vi "Trajectory Box Monitor.vi"() -> ()   [LabVIEW 2017]
uses:
  TCP/TCP Engine/Controls/RT- Queue States.ctl
  TCP/TCP Host/Controls/Control - Testscreen.ctl
  Controls/Testscreen_Input cluster.ctl
  <vilib>/addons/database/Connection.llb/Conn ObjectReference.ctl
  Controls/Network_states.ctl
  TCP/TCP Engine/TCP/TCP - Driver Control.ctl
  Variable/Global 1.vi
  <vilib>/addons/database/Connection.llb/DB Tools Open Connec (String).vi
  <vilib>/addons/database/NI_Database_API.lvlib
panel:
  out "error out":errorcluster
  out "array":string[](array[string])
  out "Test Running":bool
  in  "DataLog Duration":string="00:01:27"
  in  "Exit":bool
  in  "Report":bool
  in  "Settings":bool
  in  "Test Screen":bool
  in  "ID Status":string
  in  "?":enum32{"Option A", "Option B"}(tab)
  in  "Test Profile":T1(array[cluster])=[{"Ram Up Time"=10.0, "Hold Time"=5.0, "Ramp Down"=10.0, "Concentration Value"=25.0}, {"Ram Up Time"=15.0, "Hold Time"=10.0, "Ramp Down"=5.0, "Concentration Value"=35.0}, {"Ram Up Time"=0.0, "Hold Time"=0.0, "Ramp Down"=0.0, "Concentration Value"=0.0}]
  out "Profile Plotting":cluster{"X":dbl, "Y":dbl}[](graph)
  in  "Profile File Selection":u16(ring) items=["Test A", "Test B", "Test C"]
  in  "Iterations":dbl
  in  "Gas Selection":u16(ring) items=["Test A", "Test B", "Test C"]
  in  "Drive  2":string
  in  "Drive":string
  in  "IP Address":string
  in  "error in (no error)":errorcluster
  in  "Note":string
  in  "Tab- Main":enum32{"Settings", "Report", "Testscreen"}(tab)
  in  "Tab Control Testscreen 4":enum32{"Channel Mapping", "Test Settings"}(tab)
  in  "Channel Mapping":T2(array[cluster])
  in  "Sampling Frequency (Hz)":string="Trajectory"
  in  "Wifi Name":string="Trajectory"
  in  "Test Inactivity Time":dbl=30.0 format="%<%H:%M:%S>t"
  in  "Drive Path":path=path "D:/Trajectory Data"
  in  "cRIO IP Address":string="192.168.1.1"
  out "Test Time":dbl=1.0 format="%<%H:%M:%S>t"
  in  "Save Test Settings":bool
  in  "Tab Control Testscreen 5":enum32{"Report", "Detailed Report"}(tab)
  in  "Fetch Report":bool
  in  "To Date & Time":timestamp format="%<%x>T"
  in  "From Date & Time":timestamp format="%<%x>T"
  out "Report Data":i32(listbox)
  in  "Test Stop Time :":string="12:59:05"
  in  "Tab Control Testscreen 6":enum32{"Data", "Histogram"}(tab)
  in  "Report Data 2":i32(listbox)
  out "XY Graph 3":cluster{i32, "Numeric":u16}[](graph)
  in  "ID Status :":string="00068OK"
  in  "ID :":string="Trajectory"
  in  "Angle :":string="Multi"
  in  "Flow :":string="Flow"
  in  "Material :":string="Cole"
  in  "Furnace :":string="G Furnace"
  in  "Test Start Time:":string="12:59:05"
  in  "Date :":string="02/07/2021"
  out "Date":string
  in  "Tab- Main 2":T3(tab)
  in  "Test details":T4={"Furnace"="Furnace A", "Material"="Coke", "Angle"="Multi Angle", "ID"="Trajectory 9", "Flowrate"="Flow", "Test Name"="Coke Burn", "Tested By"="Anirban"}
  in  "Save Test Info":bool
  out "Data Logging Path":path
  in  "Probe 2":bool[](array[boolean])=[TRUE, FALSE, FALSE, FALSE, TRUE, FALSE, FALSE, FALSE, FALSE, FALSE, FALSE, FALSE, FALSE, FALSE, FALSE, FALSE, FALSE, FALSE, FALSE, FALSE, FALSE, FALSE, FALSE, FALSE, FALSE, FALSE, FALSE, FALSE, FALSE, FALSE, FALSE, FALSE, FALSE, FALSE, FALSE, FALSE, FALSE, FALSE, FALSE, FALSE, FALSE, FALSE, FALSE, FALSE, FALSE, FALSE, FALSE, FALSE, FALSE, FALSE, FALSE, FALSE, FALSE, FALSE, FALSE, FALSE, FALSE, FALSE, FALSE, FALSE]
  in  "Probe":bool[](array[boolean])
  in  "Probe 3":bool[](array[boolean])=[TRUE, FALSE, FALSE, FALSE, TRUE, FALSE, FALSE, FALSE, FALSE, FALSE, FALSE, FALSE, FALSE, FALSE, FALSE, FALSE, FALSE, FALSE, FALSE, FALSE, FALSE, FALSE, FALSE, FALSE, FALSE, FALSE, FALSE, FALSE, FALSE, FALSE, FALSE, FALSE, FALSE, FALSE, FALSE, FALSE, FALSE, FALSE, FALSE, FALSE, FALSE, FALSE, FALSE, FALSE, FALSE, FALSE, FALSE, FALSE, FALSE, FALSE, FALSE, FALSE, FALSE, FALSE, FALSE, FALSE, FALSE, FALSE, FALSE, FALSE]
  out "XY Graph":cluster{i32, "Numeric":i32}[](graph)
  in  "Setup":bool
  out "Datalog Duration":dbl format="%<%H:%M:%S>t"
  in  "Disk Space Host":string="Trajectory 9"
  in  "Disk Space cRIO":string="Trajectory 9"
  in  "Calibrations":bool
  in  "Alarms":i32(listbox)
  out "Wifi":bool=TRUE
  out "Logging 3":bool=TRUE
  in  "Start Test":bool
  in  "Stop Test":bool
  out "Message":string="Acquiring Data"
  # "Test Setup Setting"
  # "Trajectory Box Monitor System"
  # "Trajectory Box Monitor"
  # "1"
  # "5"
  # "10"
  # "15"
  # "20"
  # "41"
  # "45"
  # "50"
  # "55"
  # "60"
  # "21"
  # "25"
  # "30"
  # "40"
  # "35"
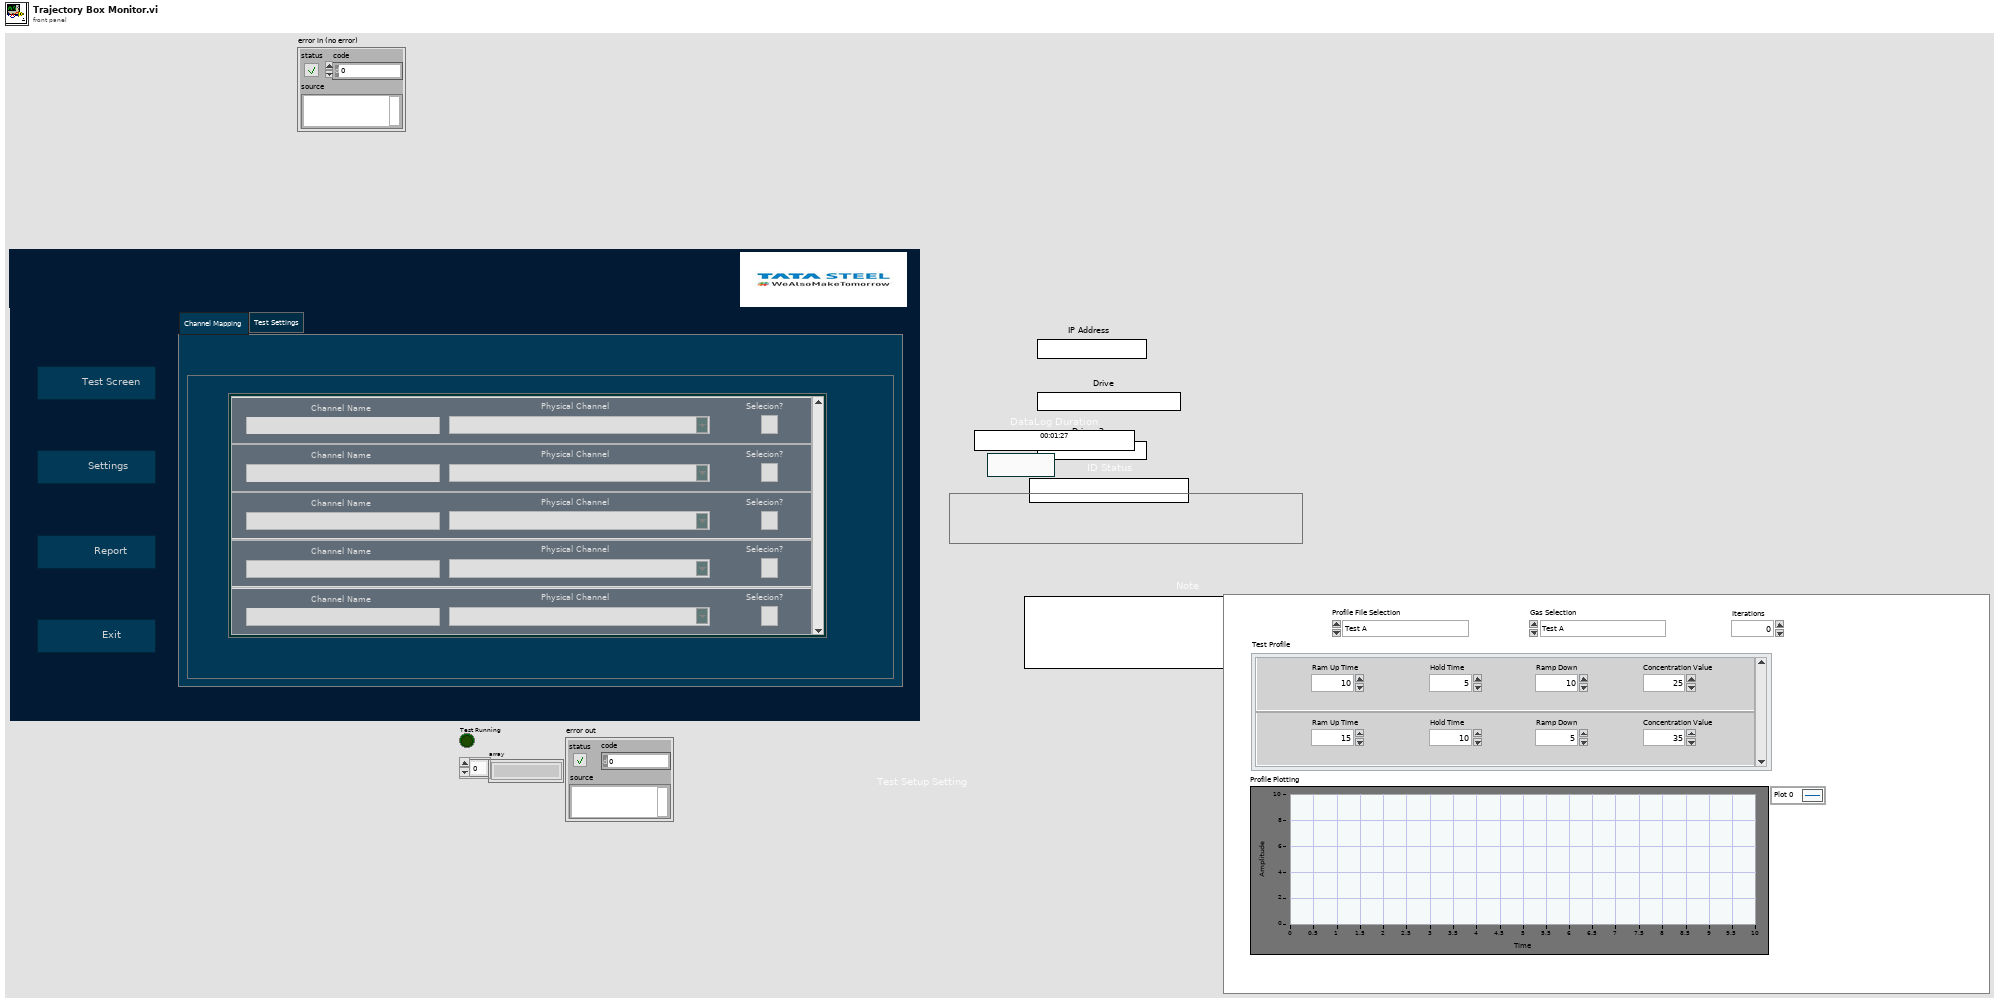
[diagram p1: front panel]
types:
  T1 = cluster{"Ram Up Time":dbl, "Hold Time":dbl, "Ramp Down":dbl, "Concentration Value":dbl}[]
  T2 = cluster{"Channel Name":string, " Physical Channel":tag, "Selecion?":bool}[]
  T3 = enum32{"Test Information", "Sensor Status", "Histogram", "Info", "Software Log"}
  T4 = cluster{"Furnace":string, "Material":string, "Angle":string, "ID":string, "Flowrate":string, "Test Name":string, "Tested By":string}
  T5 = typedef "Network_states.ctl" = enum16{"Connect", "Transfer Files", "Close"}
  T6 = typedef "Testscreen_Input cluster.ctl" = cluster{"Message":string, "Histogram Data":i32[], "Timer 1":u32, "Test Running":bool, "connection reference":T7}
  T7 = typedef "NI_Database_API.lvlib/Conn ObjectReference.ctl" = refnum<k1>
  T8 = typedef "Control - Testscreen.ctl" = enum16{"No Event", "Init", "Download Files", "Test Running", "Update Test Results", "Machine Unhealthy", "Autotest Started", "Test Aborted", "Sequence Complete", "Update Sensor Data", "Log File Available", "Machine Mode", "Aux Logging Started", "Aux File Saved", "Get PID Values", "View Report", "Exit", "Wait", "Abort", "Copy Log File", "Send Test Details"}
  T9 = typedef "RT- Queue States.ctl" = enum16{"Initialize", "Enqueue", "Enqueue Priority", "Dequeue", "Flush", "Destroy"}
  T10 = cluster{"Test details":cluster{"Furnace":string, "Material":string, "Angle":string, "ID":string, "Flowrate":string, "Test Name":string, "Tested By":string}, "Datalog Duration":dbl}
  T11 = typedef "TCP - Driver Control.ctl" = enum16{"Test Settings", "Boolean Commands", "Test Results", "Send Test Details"}
  T12 = cluster{"Channel Name":string, " Physical Channel":tag, "Selecion?":bool}
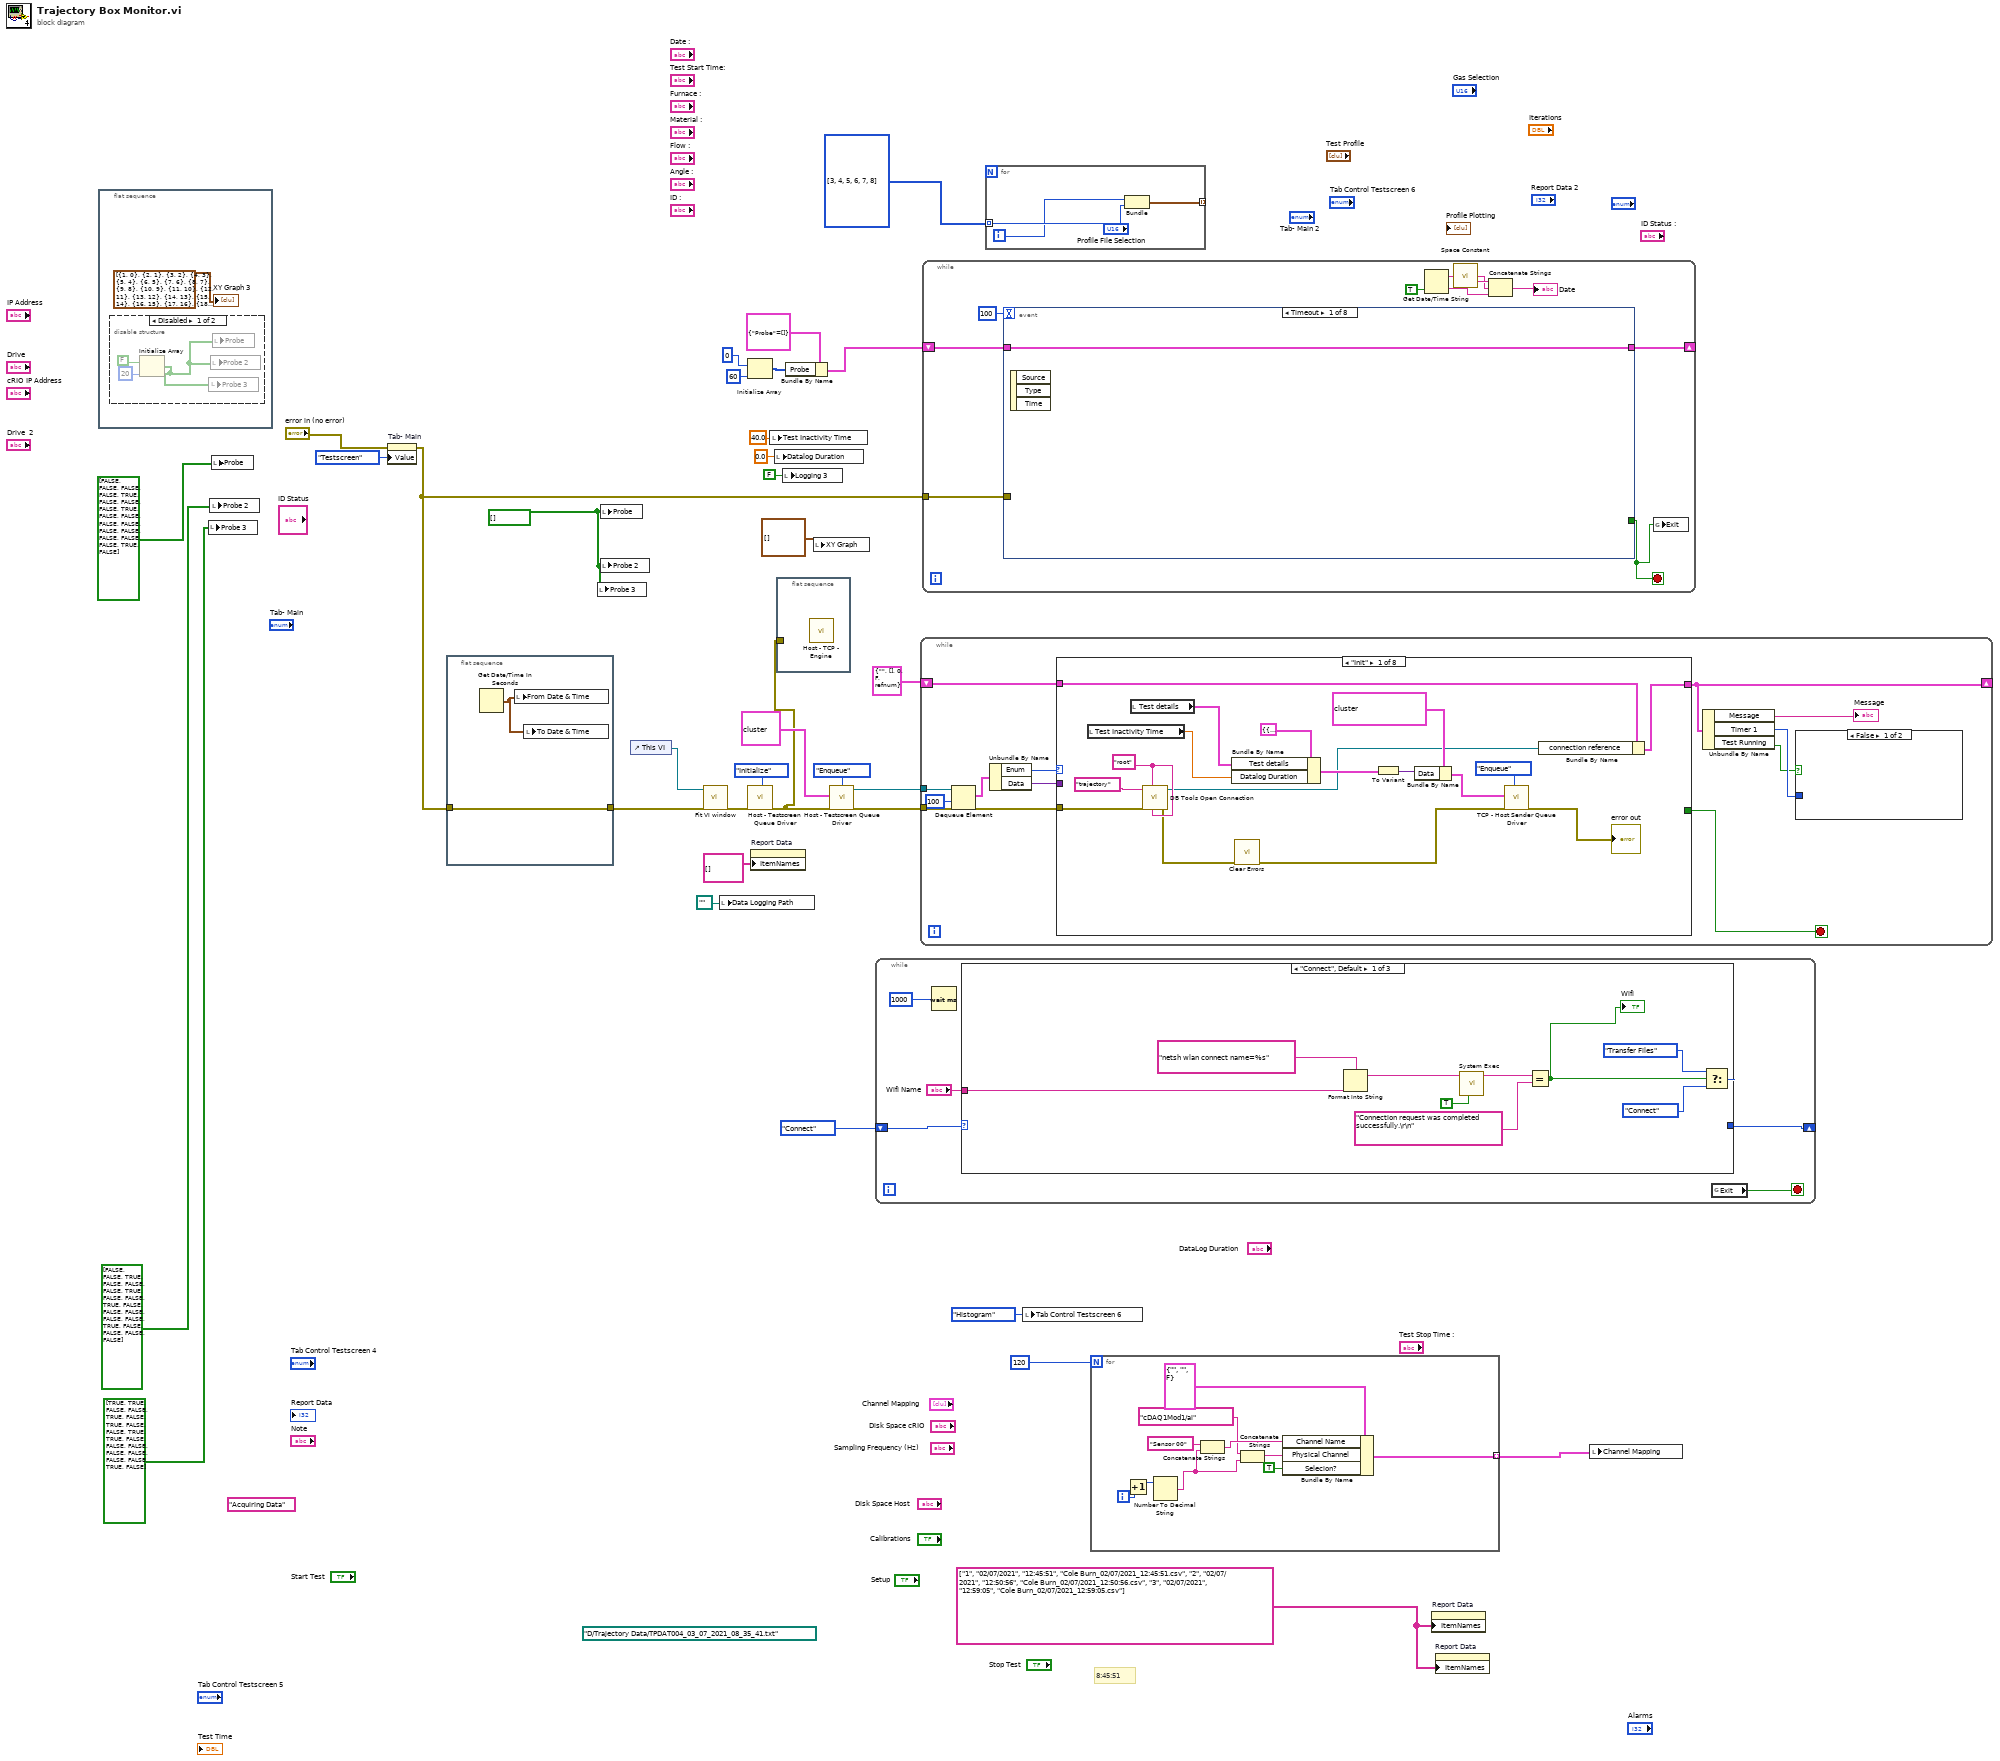
[diagram p0: block diagram]
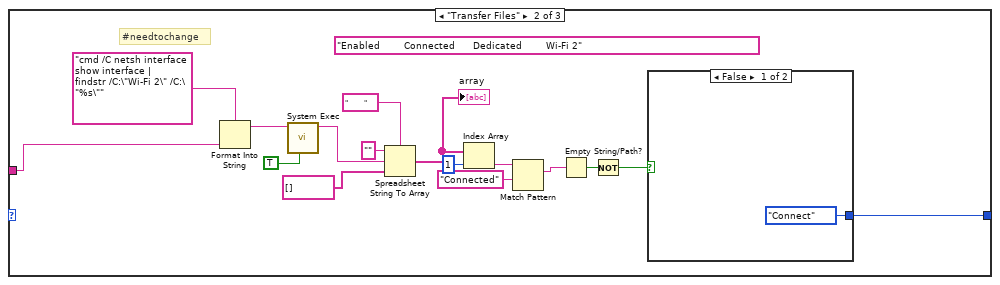
[diagram p2: hidden frame]
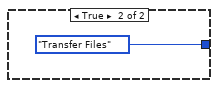
[diagram p3: hidden frame]
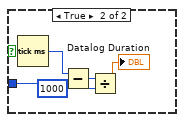
[diagram p5: hidden frame]
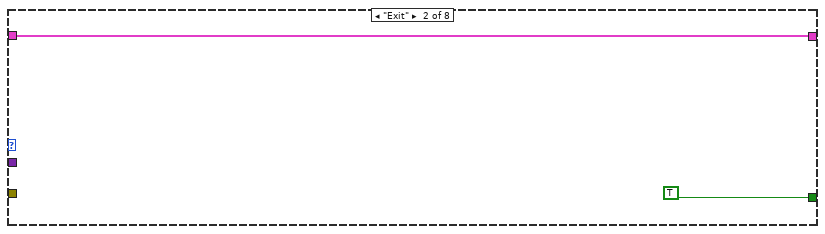
[diagram p6: hidden frame]
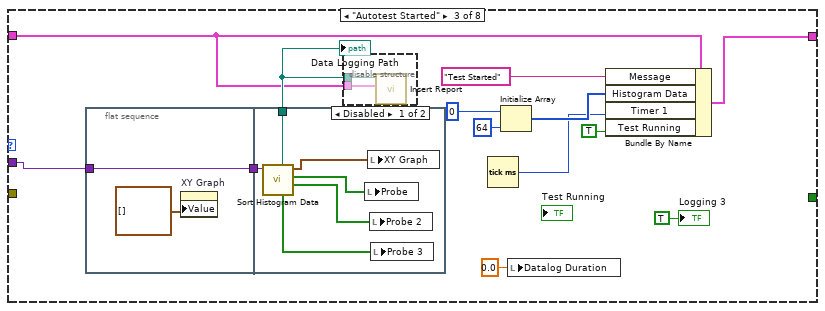
[diagram p7: hidden frame]
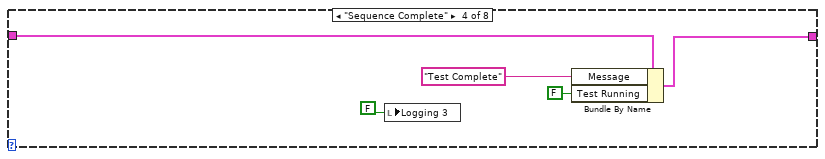
[diagram p9: hidden frame]
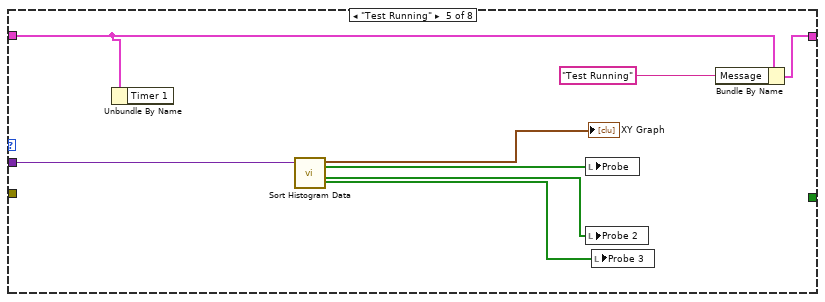
[diagram p10: hidden frame]
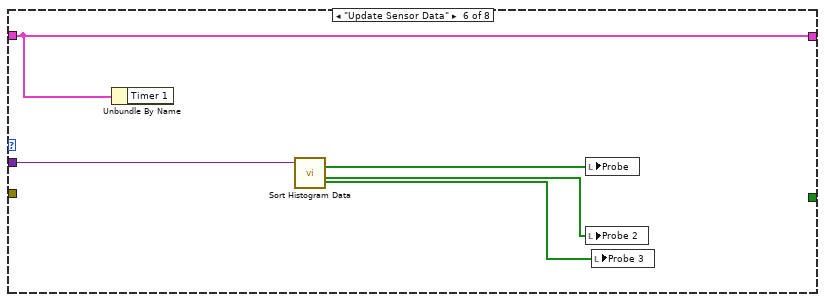
[diagram p11: hidden frame]
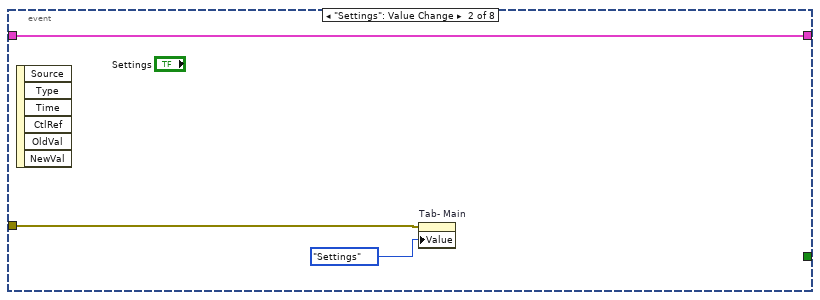
[diagram p15: hidden frame]
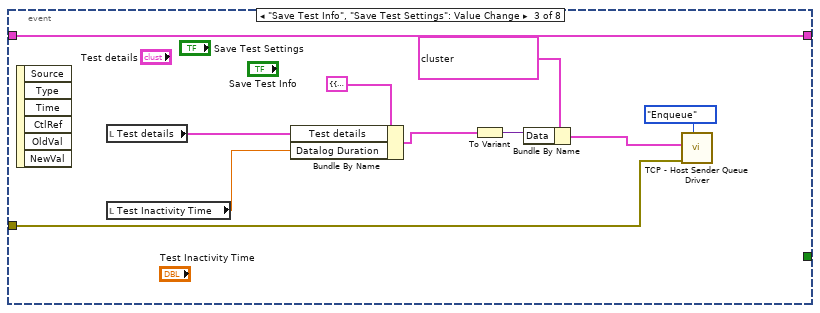
[diagram p16: hidden frame]
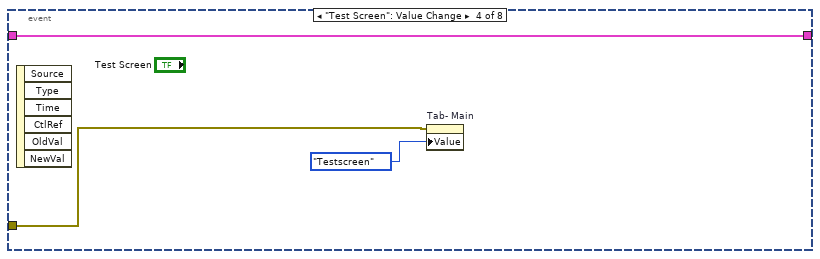
[diagram p17: hidden frame]
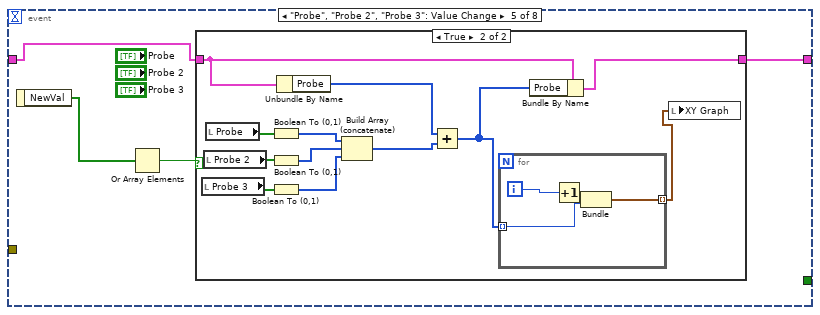
[diagram p18: hidden frame]
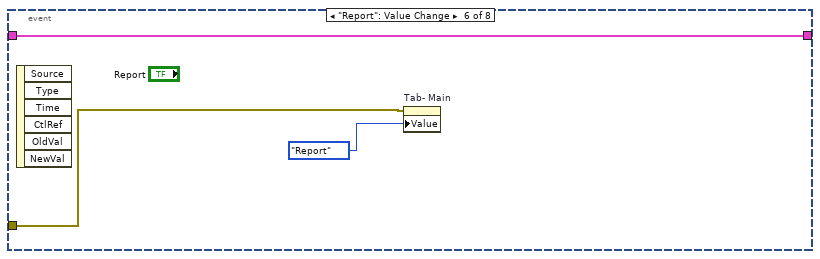
[diagram p20: hidden frame]
diagram:
  w13 = bool[] [] ("Probe")
  w20 = string[][] [["1", "02/07/2021", "12:45:51", "Cole Burn_02/07/2021_12:45:51.csv"], ["2", "02/07/2021", "12:50:56", "Cole Burn_02/07/2021_12:50:56.csv"], ["3", "02/07/2021", "12:59:05", "Cole Burn_02/07/2021_12:59:05.csv"]] ("Item Names")
  (unwired) path "D:/Trajectory Data/TPDAT004_03_07_2021_08_35_41.txt" ("Data Logging Path")
  (unwired) "Acquiring Data" ("Message")
  # "8:45:51"
  n1 = flat-sequence {
    frame #0 {
      n2 = disable-structure shown="Disabled" {
        frame Disabled {
          n3 = Initialize Array(FALSE ("Boolean"), 20 ("dimension size")) -> (w36:bool[])
          n4 = local write "Probe 3"(w36) -> ()
          n5 = local write "Probe 2"(w36) -> ()
          n6 = local write "Probe"(w36) -> ()
        }
        frame Enabled {
        }
      }
      "XY Graph 3" <- cluster{i32, "Numeric":u16}[] [{1, "Numeric"=0}, {2, "Numeric"=1}, {3, "Numeric"=2}, {4, "Numeric"=3}, {5, "Numeric"=4}, {6, "Numeric"=5}, {7, "Numeric"=6}, {8, "Numeric"=7}, {9, "Numeric"=8}, {10, "Numeric"=9}, {11, "Numeric"=10}, {12, "Numeric"=11}, {13, "Numeric"=12}, {14, "Numeric"=13}, {15, "Numeric"=14}, {16, "Numeric"=15}, {17, "Numeric"=16}, {18, "Numeric"=17}, {19, "Numeric"=18}, {20, "Numeric"=19}, {21, "Numeric"=20}, {22, "Numeric"=21}, {23, "Numeric"=22}, {24, "Numeric"=23}, {25, "Numeric"=24}, {26, "Numeric"=25}, {27, "Numeric"=26}, {28, "Numeric"=27}, {29, "Numeric"=28}, {30, "Numeric"=29}, {30, "Numeric"=29}, {31, "Numeric"=28}, {32, "Numeric"=27}, {33, "Numeric"=26}, {34, "Numeric"=25}, {35, "Numeric"=24}, {36, "Numeric"=23}, {37, "Numeric"=22}, {38, "Numeric"=21}, {39, "Numeric"=20}, {40, "Numeric"=19}, {41, "Numeric"=18}, {42, "Numeric"=17}, {43, "Numeric"=16}, {44, "Numeric"=15}, {45, "Numeric"=14}, {46, "Numeric"=13}, {47, "Numeric"=12}, {48, "Numeric"=11}, {49, "Numeric"=10}, {50, "Numeric"=9}, {51, "Numeric"=8}, {52, "Numeric"=7}, {53, "Numeric"=6}, {54, "Numeric"=5}, {55, "Numeric"=4}, {56, "Numeric"=3}, {57, "Numeric"=2}, {58, "Numeric"=1}, {59, "Numeric"=0}] ("appended array 2")
    }
  }
  n7 = local write "Probe 3"(bool[] [TRUE, TRUE, FALSE, FALSE, TRUE, FALSE, TRUE, FALSE, FALSE, TRUE, TRUE, FALSE, FALSE, FALSE, FALSE, FALSE, FALSE, FALSE, TRUE, FALSE] ("Probe")) -> ()
  n8 = local write "Probe 2"(bool[] [FALSE, FALSE, TRUE, FALSE, FALSE, FALSE, TRUE, FALSE, FALSE, TRUE, FALSE, FALSE, FALSE, FALSE, FALSE, TRUE, FALSE, FALSE, FALSE, FALSE] ("Probe")) -> ()
  n9 = local write "Probe"(bool[] [FALSE, FALSE, FALSE, FALSE, TRUE, FALSE, FALSE, FALSE, TRUE, FALSE, FALSE, FALSE, FALSE, FALSE, FALSE, FALSE, FALSE, FALSE, TRUE, FALSE] ("Probe")) -> ()
  n10 = property on="Tab- Main" class="TabCtl (strict)"(error in="error in (no error)", "Value"=enum32{"Settings", "Report", "Testscreen"}."Testscreen" ("Tab- Main")) -> (error out=w4:errorcluster)  [unwired: 1 in, 1 out]
  n11 = flat-sequence {
    tunnel: [w40] -> w3
    tunnel: w4 -> [w40]
    frame #0 {
      n12 = Get Date/Time In Seconds() -> (seconds since 1Jan1904=w39:timestamp)
      n13 = local write "From Date & Time"(w39) -> ()
      n14 = local write "To Date & Time"(w39) -> ()
    }
  }
  n15 = local write "Probe 3"(w13) -> ()
  n16 = local write "Probe"(w13) -> ()
  n17 = local write "Probe 2"(w13) -> ()
  n18 = control-ref of="This VI"() -> (w9:refnum<vi>)
  n19 = call "Fit VI window.vi"("error in (no error)"=w3, "VI Ref (calling VI)"=w9) -> ("error out"=w10:errorcluster)  [unwired: 9 in]
  n20 = local write "Data Logging Path"(path "" ("Data Logging Path")) -> ()
  n21 = Initialize Array(0 ("Numeric"), 60 ("dimension size")) -> (w30:i32[])
  n22 = call "Host - Testscreen Queue Driver.vi"("Cases"=RT-_Queue_States."Initialize", "error in (no error)"=w10) -> ("error out"=w1:errorcluster)  [unwired: 7 in, 2 out]
  n23 = property on="Report Data" class="MCListbox (strict)"("ItemNames"=string[][] [] ("Item Names")) -> ()  [unwired: 2 in, 2 out]
  n24 = local write "Test Inactivity Time"(40.0 ("Datalog Duration")) -> ()
  n25 = local write "Datalog Duration"(0.0 ("Datalog Duration")) -> ()
  n26 = flat-sequence {
    tunnel: w1 -> [_]
    frame #0 {
      n27 = call "Host - TCP - Engine.vi"() -> ()  [unwired: 12 in]
    }
  }
  n28 = local write "Logging 3"(FALSE ("Logging 3")) -> ()
  n29 = Bundle By Name(cluster=cluster{"Probe":i32[]} {"Probe"=[]}, "Probe"=w30) -> (w28:cluster{"Probe":i32[]})
  n30 = local write "XY Graph"(cluster{i32, "Numeric":i32}[] [] ("XY Graph")) -> ()
  n31 = call "Host - Testscreen Queue Driver.vi"("Cases"=RT-_Queue_States."Enqueue", "error in (no error)"=w1, "Element In"=cluster{"Data":variant, "Enum":T8} {"Data"=variant, "Enum"=enum."Init"}) -> ("error out"=w15:errorcluster, "queue out"=w17:refnum<queue>)  [unwired: 6 in, 1 out]
  n32 = while {
    shift-right: [w43] -> _
    shift-left: Network_states."Connect" -> [w44]
    stop <- w45 stop-if-true
    n33 = Wait (ms)(milliseconds to wait=u32 1000) -> ()  [unwired: 1 out]
    n34 = case shown="\"Connect\", Default" w44 {
      tunnel: [w48 w56 _] -> w43
      tunnel: "Wifi Name" -> [w47 w68 _]
      frame "Connect", Default {
        n35 = Format Into String(format string="netsh wlan connect name=%s" ("command line"), w47) -> (resulting string=w51:string)  [unwired: 2 in, 1 out]
        n36 = call <vilib>:"System Exec.vi"("run minimized? (F)"=TRUE, "command line"=w51) -> ("standard output"=w54:string)  [unwired: 6 in, 3 out]
        n37 = Equal?(x=w54, y="Connection request was completed successfully.\r\n") -> (x = y?=w46:bool)
        "Wifi" <- w46
        n38 = Select(t=Network_states."Transfer Files", s=w46, f=Network_states."Connect") -> (s? t:f=w48:T5)
      }
      frame "Transfer Files" {
        (unwired) "Enabled        Connected      Dedicated        Wi-Fi 2" ("format string")
        # "#needtochange"
        n39 = Format Into String(format string="cmd /C netsh interface show interface | findstr /C:\"Wi-Fi 2\" /C:\"%s\"" ("command line"), w68) -> (resulting string=w70:string)  [unwired: 2 in, 1 out]
        n40 = call <vilib>:"System Exec.vi"("run minimized? (F)"=TRUE, "command line"=w70) -> ("standard output"=w66:string)  [unwired: 6 in, 3 out]
        n41 = Spreadsheet String To Array(delimiter (Tab)="        ", format string="", spreadsheet string=w66, array type (2D Dbl)=string[] []) -> (array=w63:string[])
        "array" <- w63
        n42 = Index Array(array=w63, index=1) -> (element=w61:string)
        n43 = Match Pattern(string=w61, regular expression="Connected") -> (match substring=w59:string)  [unwired: 1 in, 3 out]
        n44 = Empty String/Path?(string/path=w59) -> (empty?=w58:bool)
        n45 = Not(x=w58) -> (.not. x?=w57:bool)
        n46 = case shown="False" w57 {
          tunnel: [Network_states."Connect" Network_states."Transfer Files"] -> w56
          frame False {
          }
          frame True {
          }
        }
      }
      frame "Close" {
      }
    }
    n47 = global read "Global 1.vi" "Exit"() -> (w45:bool)
  }
  n48 = while {
    tunnel: w15 -> [w84]
    tunnel: w17 -> [w85]
    shift-right: [w79] -> _
    shift-left: T6 {"Message"="", "Histogram Data"=[], "Timer 1"=0, "Test Running"=FALSE, "connection reference"=refnum} -> [w80]
    stop <- w86 stop-if-true
    n49 = Dequeue Element(queue=w85, timeout in ms (-1)=100, error in (no error)=w84) -> (element=w82:cluster{"Data":variant, "Enum":T8}, error out=w83:errorcluster)  [unwired: 2 out]
    n50 = Unbundle By Name(w82) -> ("Enum"=w81:T8, "Data"=w77:variant)
    n51 = case shown="\"Init\"" w81 {
      tunnel: w83 -> [w98 _ _ _ _ _ _ _]
      tunnel: [_ TRUE _ _ _ _ _ _] -> w86
      tunnel: w80 -> [w95 w109 w111 w138 w139 w147 w152 w153]
      tunnel: [w94 w109 w122 w136 w142 w147 w152 w153] -> w79
      tunnel: w77 -> [_ _ w118 _ w146 w151 _ _]
      frame "Init" {
        w99 = "root" ("userID")
        n52 = local read "Test Inactivity Time"() -> (w101:dbl)
        n53 = local read "Test details"() -> (w103:T4)
        n54 = call-poly <vilib>:"DB Tools Open Connection.vi"("password"=w99, "userID"=w99, "error in (no error)"=w98, "connection information"="trajectory") -> ("error out"=w97:errorcluster, "connection reference"=w96:T7)  [unwired: 4 in]
        n55 = Bundle By Name(cluster=T10 {"Test details"={"Furnace"="Furnace A", "Material"="Aluminium", "Angle"="Multi Angle", "ID"="Trajectory 9", "Flowrate"="Flow", "Test Name"="Coke Burn", "Tested By"="Anirban"}, "Datalog Duration"=0.0}, "Test details"=w103, "Datalog Duration"=w101) -> (w102:T10)
        n56 = call <vilib>:"Clear Errors.vi"("error in (no error)"=w97) -> ("error out"=w93:errorcluster)  [unwired: 5 in, 1 out]
        n57 = To Variant(anything=w102) -> (Variant=w105:variant)
        n58 = Bundle By Name(cluster=cluster{"Data":variant, "State":T11} {"Data"=variant, "State"=enum."Send Test Details"} ("Element In"), "Data"=w105) -> (w108:cluster{"Data":variant, "State":T11})
        n59 = call "TCP - Host Sender Queue Driver.vi"("Cases"=RT-_Queue_States."Enqueue", "error in (no error)"=w93, "Element In"=w108) -> ("error out"=→"error out":errorcluster)  [unwired: 6 in, 2 out]
        n60 = Bundle By Name(cluster=w95, "connection reference"=w96) -> (w94:T6)
      }
      frame "Exit" {
      }
      frame "Autotest Started" {
        n61 = flat-sequence {
          tunnel: w118 -> [w127]
          tunnel: [w127] -> w117
          tunnel: w117 -> [w133]
          tunnel: [w128] -> w112
          frame #0 {
            n62 = property on="XY Graph" class="XYGraph (strict)"("Value"=cluster{i32, "Numeric":u16}[] [] ("XY Graph")) -> ()  [unwired: 2 in, 2 out]
          }
          frame #1 {
            n63 = call "Sort Histogram Data.vi"("Data"=w133) -> ("Array 2"=w130:bool[], "Array 3"=w131:bool[], "XY Graph"=w132:cluster{i32, "Numeric":i32}[], "Array"=w129:bool[], "File Path"=w128:path)  [unwired: 6 in]
            n64 = local write "Probe"(w131) -> ()
            n65 = local write "XY Graph"(w132) -> ()
            n66 = local write "Probe 2"(w130) -> ()
            n67 = local write "Probe 3"(w129) -> ()
          }
        }
        n68 = disable-structure shown="Disabled" {
          disable-tunnel: w112 -> [w125 _]
          disable-tunnel: w111 -> [w124 _]
          frame Disabled {
            n69 = call "Insert Report.vi"("Cluster"=w124, "Path"=w125) -> ()  [unwired: 9 in, 1 out]
          }
          frame Enabled {
          }
        }
        n70 = Tick Count (ms)() -> (millisecond timer value=w116:u32)
        n71 = Initialize Array(0, 64 ("dimension size")) -> (w119:i32[])
        n72 = local write "Datalog Duration"(0.0 ("Datalog Duration")) -> ()
        n73 = Bundle By Name(cluster=w111, "Message"="Test Started", "Histogram Data"=w119, "Timer 1"=w116, "Test Running"=TRUE) -> (w122:T6)
        "Data Logging Path" <- w112
        "Logging 3" <- TRUE ("Logging 3")
      }
      frame "Sequence Complete" {
        n74 = local write "Logging 3"(FALSE ("Logging 3")) -> ()
        n75 = Bundle By Name(cluster=w138, "Message"="Test Complete", "Test Running"=FALSE) -> (w136:T6)
      }
      frame "Test Running" {
        n76 = Unbundle By Name(w139) -> ()  [unwired: 1 out]
        n77 = call "Sort Histogram Data.vi"("Data"=w146) -> ("Array 2"=w144:bool[], "Array 3"=w145:bool[], "XY Graph"=→"XY Graph":cluster{i32, "Numeric":i32}[], "Array"=w143:bool[])  [unwired: 6 in, 1 out]
        n78 = local write "Probe"(w145) -> ()
        n79 = local write "Probe 2"(w144) -> ()
        n80 = local write "Probe 3"(w143) -> ()
        n81 = Bundle By Name(cluster=w139, "Message"="Test Running") -> (w142:T6)
      }
      frame "Update Sensor Data" {
        n82 = Unbundle By Name(w147) -> ()  [unwired: 1 out]
        n83 = call "Sort Histogram Data.vi"("Data"=w151) -> ("Array 2"=w149:bool[], "Array 3"=w150:bool[], "Array"=w148:bool[])  [unwired: 6 in, 2 out]
        n84 = local write "Probe"(w150) -> ()
        n85 = local write "Probe 2"(w149) -> ()
        n86 = local write "Probe 3"(w148) -> ()
      }
      frame "No Event", Default {
      }
      frame "Update Test Results" {
      }
    }
    n87 = Unbundle By Name(w79) -> ("Message"=→"Message":string, "Timer 1"=w76:u32, "Test Running"=w75:bool)
    n88 = case shown="False" w75 {
      tunnel: w76 -> [_ w90]
      frame False {
      }
      frame True {
        n89 = Tick Count (ms)() -> (millisecond timer value=w91:u32)
        n90 = Subtract(x=w91, y=w90) -> (x-y=w89:u32)
        n91 = Divide(x=w89, y=u32 1000) -> (x/y=→"Datalog Duration":dbl)
      }
    }
  }
  n92 = while {
    tunnel: w4 -> [w163]
    shift-right: [w161] -> _
    shift-left: w28 -> [w162]
    stop <- w154 stop-if-true
    n93 = event shown="[0] Timeout" {
      selector: _ -> [_ _ _ _ _ _ _ _]
      dyn-events: _ -> [_ _ _ _ _ _ _ _]
      timeout: 100 -> [_ _ _ _ _ _ _ _]
      tunnel: [_ _ _ _ _ _ TRUE _] -> w154
      tunnel: w163 -> [_ w167 w168 w180 _ w204 w205 _]
      tunnel: w162 -> [w164 w166 w177 w179 w182 w203 w208 w212]
      tunnel: [w164 w166 w177 w179 w181 w203 w208 w212] -> w161
      event Timeout {
        n94 = event-data() -> ()  [unwired: 1 in, 3 out]
      }
      event "Settings": Value Change {
        n95 = event-data() -> ()  [unwired: 1 in, 6 out]
        n96 = property on="Tab- Main" class="TabCtl (strict)"(error in=w167, "Value"=enum32{"Settings", "Report", "Testscreen"}."Settings" ("Tab- Main")) -> ()  [unwired: 1 in, 2 out]
      }
      event "Save Test Info", "Save Test Settings": Value Change {
        n97 = event-data() -> ()  [unwired: 1 in, 6 out]
        n98 = local read "Test details"() -> (w174:T4)
        n99 = local read "Test Inactivity Time"() -> (w176:dbl)
        n100 = Bundle By Name(cluster=T10 {"Test details"={"Furnace"="Furnace A", "Material"="Aluminium", "Angle"="Multi Angle", "ID"="Trajectory 9", "Flowrate"="Flow", "Test Name"="Coke Burn", "Tested By"="Anirban"}, "Datalog Duration"=0.0}, "Test details"=w174, "Datalog Duration"=w176) -> (w175:T10)
        n101 = To Variant(anything=w175) -> (Variant=w172:variant)
        n102 = Bundle By Name(cluster=cluster{"Data":variant, "State":T11} {"Data"=variant, "State"=enum."Send Test Details"} ("Element In"), "Data"=w172) -> (w169:cluster{"Data":variant, "State":T11})
        n103 = call "TCP - Host Sender Queue Driver.vi"("Cases"=RT-_Queue_States."Enqueue", "error in (no error)"=w168, "Element In"=w169) -> ()  [unwired: 6 in, 3 out]
      }
      event "Test Screen": Value Change {
        n104 = event-data() -> ()  [unwired: 1 in, 6 out]
        n105 = property on="Tab- Main" class="TabCtl (strict)"(error in=w180, "Value"=enum32{"Settings", "Report", "Testscreen"}."Testscreen" ("Tab- Main")) -> ()  [unwired: 1 in, 2 out]
      }
      event "Probe", "Probe 2", "Probe 3": Value Change {
        n106 = event-data() -> ("NewVal"=w184:bool[])  [unwired: 1 in]
        n107 = Or Array Elements(Boolean array=w184) -> (logical OR=w183:bool)
        n108 = case shown="True" w183 {
          tunnel: w182 -> [w185 w188]
          tunnel: [w185 w187] -> w181
          frame False {
          }
          frame True {
            n109 = local read "Probe 3"() -> (w195:bool[])
            n110 = local read "Probe 2"() -> (w196:bool[])
            n111 = local read "Probe"() -> (w197:bool[])
            n112 = Boolean To (0,1)(Boolean=w197) -> (0, 1=w194:i16[])
            n113 = Boolean To (0,1)(Boolean=w196) -> (0, 1=w193:i16[])
            n114 = Boolean To (0,1)(Boolean=w195) -> (0, 1=w192:i16[])
            n115 = Unbundle By Name(w188) -> ("Probe"=w191:i32[])
            n116 = Build Array (concatenate)(w194, w193, w192) -> (w190:i16[])
            n117 = Add(x=w191, y=w190) -> (x+y=w186:i32[])
            n118 = for {
              tunnel: [w201] -> w189 mode=indexing
              tunnel: w186 -> [w200] mode=indexing
              i -> [w199]
              n119 = Increment(x=w199) -> (x+1=w198:i32)
              n120 = Bundle(w198, w200) -> (w201:cluster{i32, i32})  [unwired: 1 in]
            }
            n121 = Bundle By Name(cluster=w188, "Probe"=w186) -> (w187:cluster{"Probe":i32[]})
            n122 = local write "XY Graph"(w189) -> ()
          }
        }
      }
      event "Report": Value Change {
        n123 = event-data() -> ()  [unwired: 1 in, 6 out]
        n124 = property on="Tab- Main" class="TabCtl (strict)"(error in=w204, "Value"=enum32{"Settings", "Report", "Testscreen"}."Report" ("Tab- Main")) -> ()  [unwired: 1 in, 2 out]
      }
      event "Exit": Value Change {
        n125 = event-data() -> ()  [unwired: 1 in, 6 out]
        n126 = call "Host - Testscreen Queue Driver.vi"("Cases"=RT-_Queue_States."Enqueue", "error in (no error)"=w205, "Element In"=cluster{"Data":variant, "Enum":T8} {"Data"=variant, "Enum"=enum."Exit"}) -> ()  [unwired: 6 in, 3 out]
      }
      event "Fetch Report": Value Change {
        n127 = event-data() -> ()  [unwired: 1 in, 6 out]
        n128 = List Folder(path="Drive Path") -> (filenames=w210:string[])  [unwired: 3 in, 3 out]
        n129 = for {
          tunnel: "Drive Path" -> [w219]
          tunnel: w210 -> [w214] mode=indexing
          tunnel: [w214] -> _ mode=indexing if=w213
          n130 = Build Path(base path=w219, name or relative path=w214) -> (appended path=w218:path)
          n131 = File/Directory Info(path=w218) -> (last mod=w217:timestamp)  [unwired: 1 in, 6 out]
          n132 = In Range and Coerce(upper limit="To Date & Time", x=w217, lower limit="From Date & Time") -> (In Range?=w213:bool)  [unwired: 1 out]
        }
      }
    }
    n133 = Get Date/Time String(want seconds? (F)=TRUE) -> (date string=w158:string, time string=w156:string)  [unwired: 2 in]
    n134 = call <vilib>:"Space Constant.vi"() -> ("String"=w157:string)
    n135 = Concatenate Strings(w158, w157, w156) -> (→"Date":string)
    n136 = global write "Global 1.vi" "Exit"(w154) -> ()
  }
  n137 = for {
    tunnel: [w222] -> _ mode=indexing
    tunnel: u16[] [3, 4, 5, 6, 7, 8] -> [w221] mode=indexing
    i -> [w220]
    n138 = Bundle(w220, "Numeric"=w221) -> (w222:cluster{i32, "Numeric":u16})  [unwired: 1 in]
  }
  n139 = local write "Tab Control Testscreen 6"(enum32{"Data", "Histogram"}."Histogram" ("Tab Control Testscreen 6")) -> ()
  n140 = for {
    N: 120 -> [_]
    tunnel: [w223] -> w22 mode=indexing
    i -> [w230]
    n141 = Increment(x=w230) -> (x+1=w226:i32)
    n142 = Number To Decimal String(number=w226) -> (decimal integer string=w227:string)  [unwired: 1 in]
    n143 = Concatenate Strings("Sensor 00" ("string"), w227) -> (w229:string)
    n144 = Concatenate Strings("cDAQ1Mod1/ai" ("string"), w227) -> (w225:string)
    n145 = Bundle By Name(cluster=T12 {"Channel Name"="", " Physical Channel"="", "Selecion?"=FALSE} ("Channel Mapping"), "Channel Name"=w229, "Physical Channel"=w225, "Selecion?"=TRUE) -> (w223:T12)
  }
  n146 = property on="Report Data" class="MCListbox (strict)"("ItemNames"=w20) -> ()  [unwired: 2 in, 2 out]
  n147 = property on="Report Data" class="MCListbox (strict)"("ItemNames"=w20) -> ()  [unwired: 2 in, 2 out]
  n148 = local write "Channel Mapping"(w22) -> ()
